vi "Tosca-Start MATLAB Thread.vi"(0 "MATLAB notifier":refnum<notifier>) -> (15 "error out":errorcluster)   [LabVIEW 2020]
uses:
  Typedefs/Tosca-MATLAB Queue Data.ctl
panel:
  # "Starting MATLAB server..."
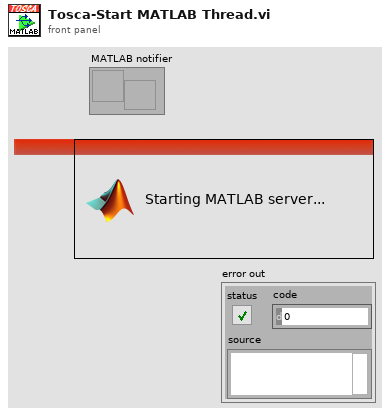
[diagram p1: front panel]
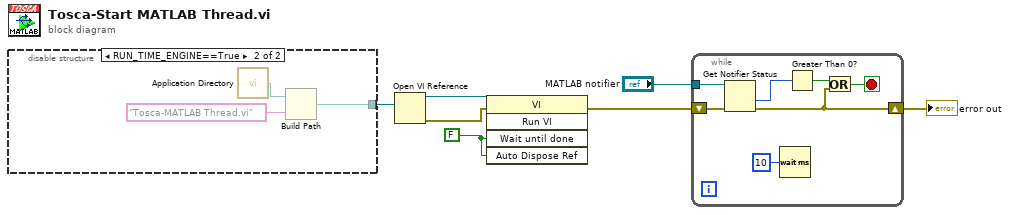
[diagram p0: block diagram]
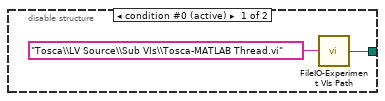
[diagram p2: hidden frame]
diagram:
  w7 = FALSE ("Wait Until Done")
  n1 = disable-structure shown="RUN_TIME_ENGINE==True" {
    disable-tunnel: [w8 w10] -> w1
    frame condition #0 (active) {
      n2 = call "FileIO-Experiment VIs Path.vi"("relpath"="Tosca\\LV Source\\Sub VIs\\Tosca-MATLAB Thread.vi") -> ("full path"=w8:path)  [unwired: 4 in]
    }
    frame condition #1 {
      n3 = call <vilib>:"Application Directory.vi"() -> ("Application Directory"=w11:path)
      n4 = Build Path(base path=w11, name or relative path="Tosca-MATLAB Thread.vi") -> (appended path=w10:path)
    }
  }
  n5 = Open VI Reference(vi path=w1) -> (vi reference=w6:refnum<vi>, error out=w5:errorcluster)  [unwired: 5 in]
  n6 = invoke class="VI" method="Run VI"(reference=w6, error in=w5, "Wait until done"=w7, "Auto Dispose Ref"=w7) -> (error out=w4:errorcluster)  [unwired: 1 in, 4 out]
  n7 = while {
    tunnel: "MATLAB notifier" -> [w19]
    shift-right: [w13] -> w2
    shift-left: w4 -> [w15]
    stop <- w14 stop-if-true
    n8 = Get Notifier Status(notifier=w19, error in (no error)=w15) -> (# waiting=w18:i32, error out=w13:errorcluster)  [unwired: 3 out]
    n9 = Wait (ms)(milliseconds to wait=u32 10) -> ()  [unwired: 1 out]
    n10 = Greater Than 0?(x=w18) -> (x > 0?=w17:bool)
    n11 = Or(x=w17, y=w13) -> (x .or. y?=w14:bool)
  }
  "error out" <- w2
